vi "_PC_Pub_Timestamp_ToString.vi"(8 "error in":errorcluster, 11 "Timestamp":timestamp) -> (0 "error out":errorcluster, 3 "Timestring":string)   [LabVIEW 2018]
doc: "%I:%M:%S%3u %p%m%d%Y"
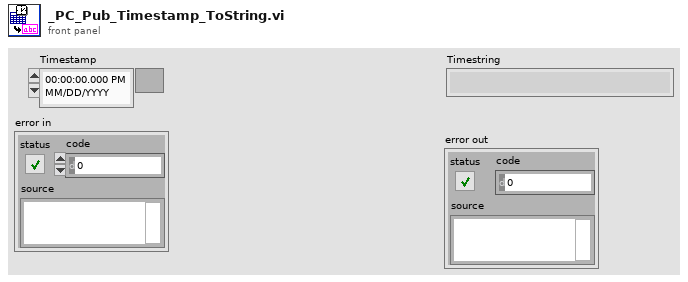
[diagram p1: front panel]
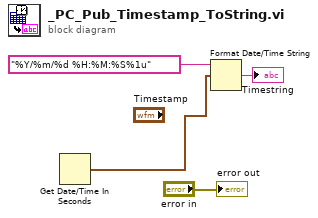
[diagram p0: block diagram]
diagram:
  n1 = Get Date/Time In Seconds() -> (seconds since 1Jan1904=w1:timestamp)
  n2 = Format Date/Time String(time format string (%c)="%Y/%m/%d %H:%M:%S%1u", seconds (now)=w1) -> (date/time string=→"Timestring":string)  [unwired: 1 in]
  "error out" <- "error in"
